vi "_PC_Spectrafilter set_rectangle_position.vi"(8 "error in (no error)":errorcluster, 10 "Coords":T1, 11 "xy graph ref":refnum<vi>) -> (0 "error out":errorcluster)   [LabVIEW 2016]
uses:
  <vilib>/Utility/miscctls.llb/LVPoint32TypeDef.ctl
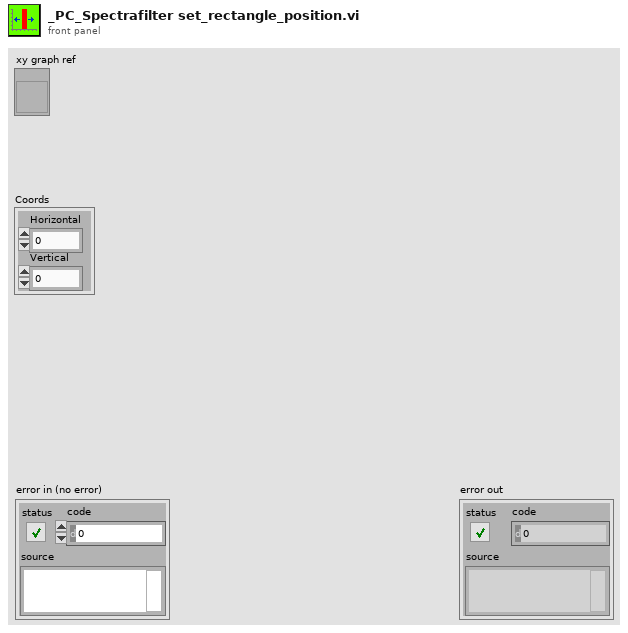
[diagram p1: front panel]
types:
  T1 = typedef "LVPoint32TypeDef.ctl" = cluster{"Horizontal":i32, "Vertical":i32}
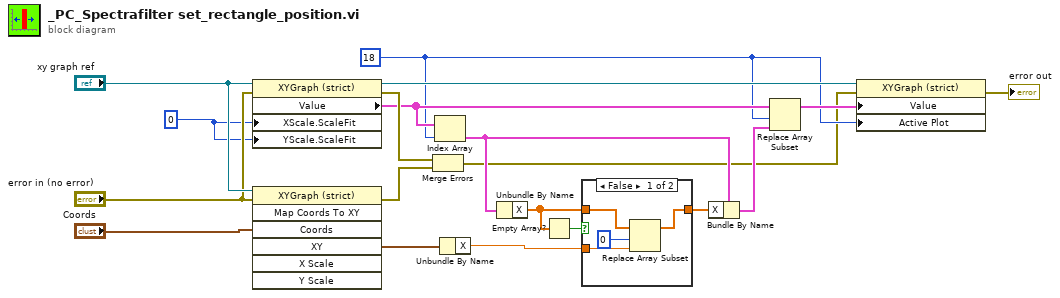
[diagram p0: block diagram]
diagram:
  w1 = u8 0 ("X Scale.Scale Fit")
  w6 = 18 ("index")
  n1 = property class="XYGraph (strict)"(reference="xy graph ref", error in="error in (no error)", "XScale.ScaleFit"=w1, "YScale.ScaleFit"=w1) -> (reference out=w17:refnum<vi>, error out=w15:errorcluster, "Value"=w9:cluster{"X":dbl[], "Y":sgl[]}[])
  n2 = invoke class="XYGraph (strict)" method="Map Coords To XY"(reference="xy graph ref", error in="error in (no error)", "Coords"="Coords") -> (error out=w16:errorcluster, "XY"=w14:cluster{"X":dbl, "Y":dbl})  [unwired: 4 in, 5 out]
  n3 = Merge Errors(w15, w16) -> (w2:errorcluster)
  n4 = Index Array(array=w9, index=w6) -> (element=w11:cluster{"X":dbl[], "Y":sgl[]})
  n5 = Unbundle By Name(w14) -> ("X"=w12:dbl)
  n6 = Unbundle By Name(w11) -> ("X"=w3:dbl[])
  n7 = Empty Array?(array=w3) -> (empty?=w4:bool)
  n8 = case shown="False" w4 {
    tunnel: w12 -> [w22 _]
    tunnel: [w21 w24] -> w10
    tunnel: w3 -> [w20 w24]
    frame False {
      n9 = Replace Array Subset(array=w20, new element=w22, index=0) -> (w21:dbl[])
    }
    frame True {
    }
  }
  n10 = Bundle By Name(cluster=w11, "X"=w10) -> (w8:cluster{"X":dbl[], "Y":sgl[]})
  n11 = Replace Array Subset(array=w9, new element=w8, index=w6) -> (w7:cluster{"X":dbl[], "Y":sgl[]}[])
  n12 = property class="XYGraph (strict)"(reference=w17, error in=w2, "Value"=w7, "Active Plot"=w6) -> (error out=→"error out":errorcluster)  [unwired: 1 out]
